vi "PH_PPMA_PowerUnit.calc Status.vi"(0 "i ref in":refnum<vi>, 5 "error in (no error)":errorcluster) -> (14 "i ref out":refnum<vi>, 19 "error out":errorcluster)   [LabVIEW 2014, in "PH_PPMA_PowerUnit.lvlib"]
doc: "This VI checks wether one of the subsystems is in failure or alarm status, if there is no information about the system or whether systems are off. It writes the information to own attributes, the GUI and publishes it as DIM service."
uses:
  PH_PPMA_PowerUnit.lvlib
  PH_StatusHandler/PH_StatusHandler.Status.ctl
  PH_StatusHandler/PH_StatusHandler.lvlib
  PH_PowerUnit_BaseClass/PH_PowerUnit_BaseClass.lvlib
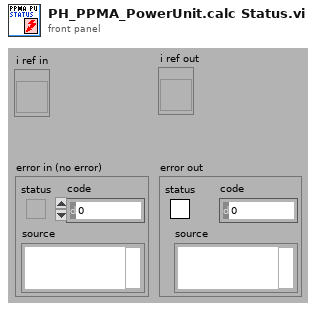
[diagram p1: front panel]
types:
  T1 = typedef "PH_StatusHandler.lvlib/PH_StatusHandler.Status.ctl" = i16
  T2 = typedef "PH_PPMA_PowerUnit.lvlib/PH_PPMA_PowerUnit.i attribute.ctl" = cluster{"GUI Refs":cluster{"Rods":refnum<vi>, "Ignitron":refnum<vi>, "Rossrelais":refnum<vi>, "Set Voltage":refnum<vi>, "PSU":refnum<vi>, "EOC":refnum<vi>, "Trigger":refnum<vi>}, "Rods":T3, "PSU":T4, "Ross Relais":T5, "Ignitron":T6, "Trigger":cluster{"State Device":T1, "linked?":bool}, "Timing Settings":cluster{"Prdc Fast?":bool, "Default Value Periodic Interval":i32, "Mercury on since":dbl, "Warm up Time Mercury [s]":dbl}, "Set Voltage [V]":dbl}
  T3 = typedef "PH_PPMA_PowerUnit.lvlib/PH_PPMA_PowerUnit.Rods Attributes.ctl" = cluster{"Instancename":string, "Device Status":T1, "linked?":bool}
  T4 = typedef "PH_PP_Common.lvlib/PH_PP_Common.PSU Attributes.ctl" = cluster{"lower limit [V]":dbl, "upper limit [V]":dbl, "Voltage set":bool, "State Device":T1, "linked?":bool}
  T5 = typedef "PH_PP_Common.lvlib/PH_PP_Common.Ross Relais Attributes.ctl" = cluster{"State Device":T1, "linked?":bool}
  T6 = typedef "PH_PP_Common.lvlib/PH_PP_Common.Ignitron Attributes.ctl" = cluster{"State Device":T1, "linked?":bool}
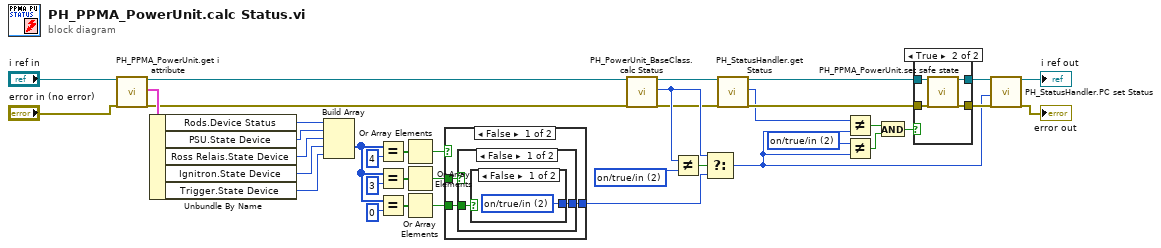
[diagram p0: block diagram]
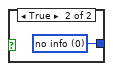
[diagram p2: hidden frame]
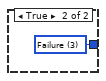
[diagram p3: hidden frame]
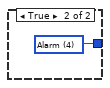
[diagram p4: hidden frame]
diagram:
  w7 = T1 2 items=["no info", "off/false/out", "on/true/in", "Failure", "Alarm", "Status 1", "Status 2", "Status 3"] ("Device Status")
  w14 = T1 2 items=["no info", "off/false/out", "on/true/in", "Failure", "Alarm", "Status 1", "Status 2", "Status 3"] ("y")
  n1 = call "PH_PPMA_PowerUnit.get i attribute.vi"("i ref in"="i ref in", "error in (no error)"="error in (no error)") -> ("i ref out"=w16:refnum<vi>, "i attribute"=w38:T2, "error out"=w23:errorcluster)  [unwired: 15 in]
  n2 = Unbundle By Name(w38) -> ("Rods.Device Status"=w24:T1, "PSU.State Device"=w37:T1, "Ross Relais.State Device"=w36:T1, "Ignitron.State Device"=w2:T1, "Trigger.State Device"=w35:T1)
  n3 = Build Array(w24, w37, w36, w2, w35) -> (w25:T1[])
  n4 = Equal?(x=w25, y=4) -> (x = y?=w33:bool[])
  n5 = Equal?(x=w25, y=3) -> (x = y?=w31:bool[])
  n6 = Equal?(x=w25, y=0) -> (x = y?=w29:bool[])
  n7 = Or Array Elements(Boolean array=w33) -> (logical OR=w28:bool)
  n8 = Or Array Elements(Boolean array=w31) -> (logical OR=w27:bool)
  n9 = Or Array Elements(Boolean array=w29) -> (logical OR=w26:bool)
  n10 = case shown="False" w28 {
    tunnel: [w41 w47] -> w3
    tunnel: w27 -> [w40 _]
    tunnel: w26 -> [w39 _]
    frame False {
      n11 = case shown="False" w40 {
        tunnel: [w43 w46] -> w41
        tunnel: w39 -> [w42 _]
        frame False {
          n12 = case shown="False" w42 {
            tunnel: [w44 w45] -> w43
            frame False {
              w44 = T1 2 items=["no info", "off/false/out", "on/true/in", "Failure", "Alarm", "Status 1", "Status 2", "Status 3"] ("Device Status")
            }
            frame True {
              w45 = T1 0 items=["no info", "off/false/out", "on/true/in", "Failure", "Alarm", "Status 1", "Status 2", "Status 3"] ("Device Status")
            }
          }
        }
        frame True {
          w46 = T1 3 items=["no info", "off/false/out", "on/true/in", "Failure", "Alarm", "Status 1", "Status 2", "Status 3"] ("Device Status")
        }
      }
    }
    frame True {
      w47 = T1 4 items=["no info", "off/false/out", "on/true/in", "Failure", "Alarm", "Status 1", "Status 2", "Status 3"] ("Device Status")
    }
  }
  n13 = call "PH_PowerUnit_BaseClass.calc Status.vi"("VI in"=w16, "error in (no error)"=w23) -> ("VI out"=w11:refnum<vi>, "PU Status"=w13:T1, "error out"=w9:errorcluster)  [unwired: 15 in]
  n14 = Not Equal?(x=w13, y=w14) -> (x != y?=w15:bool)
  n15 = Select(t=w13, s=w15, f=w3) -> (s? t:f=w6:T1)
  n16 = call "PH_StatusHandler.get Status.vi"("VI in"=w11, "error in"=w9) -> ("VI out"=w10:refnum<vi>, "Status"=w1:T1, "error out"=w8:errorcluster)  [unwired: 15 in]
  n17 = Not Equal?(x=w1, y=w6) -> (x != y?=w12:bool)
  n18 = Not Equal?(x=w7, y=w6) -> (x != y?=w5:bool)
  n19 = And(x=w12, y=w5) -> (x .and. y?=w4:bool)
  n20 = case shown="True" w4 {
    tunnel: w10 -> [w49 w53]
    tunnel: w8 -> [w48 w52]
    tunnel: [w49 w51] -> w19
    tunnel: [w48 w50] -> w20
    frame False {
    }
    frame True {
      n21 = call "PH_PPMA_PowerUnit.set safe state.vi"("i ref in"=w53, "error in (no error)"=w52) -> ("i ref out"=w51:refnum<vi>, "error out"=w50:errorcluster)  [unwired: 16 in]
    }
  }
  n22 = call "PH_StatusHandler.PC set Status.vi"("i ref in"=w19, "Status"=w6, "error in (no error)"=w20) -> ("i ref out"=→"i ref out":refnum<vi>, "error out"=→"error out":errorcluster)  [unwired: 15 in]
